vi "BRig_Host_formatData_test3_p2_subunit1.vi"(7 "input_filePath":string, 8 "input_error":errorcluster, 9 "input_data":u16[][](array[numeric]), 10 "input_headers":string[](array[string]), 11 "input_hdl_Workbooks":refnum<k7>) -> (0 "output_error":errorcluster, 3 "output_hdl_Worksbooks":refnum<k7>)   [LabVIEW 2014]
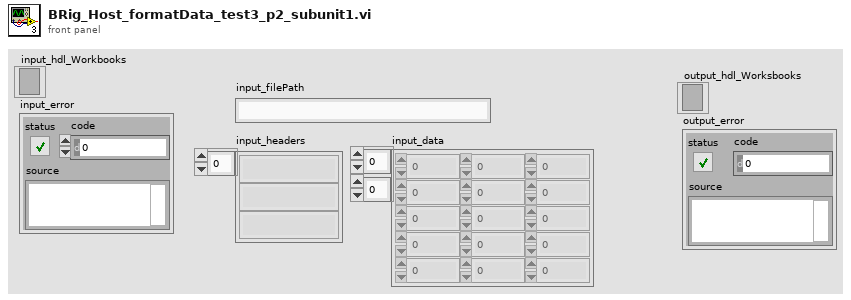
[diagram p1: front panel]
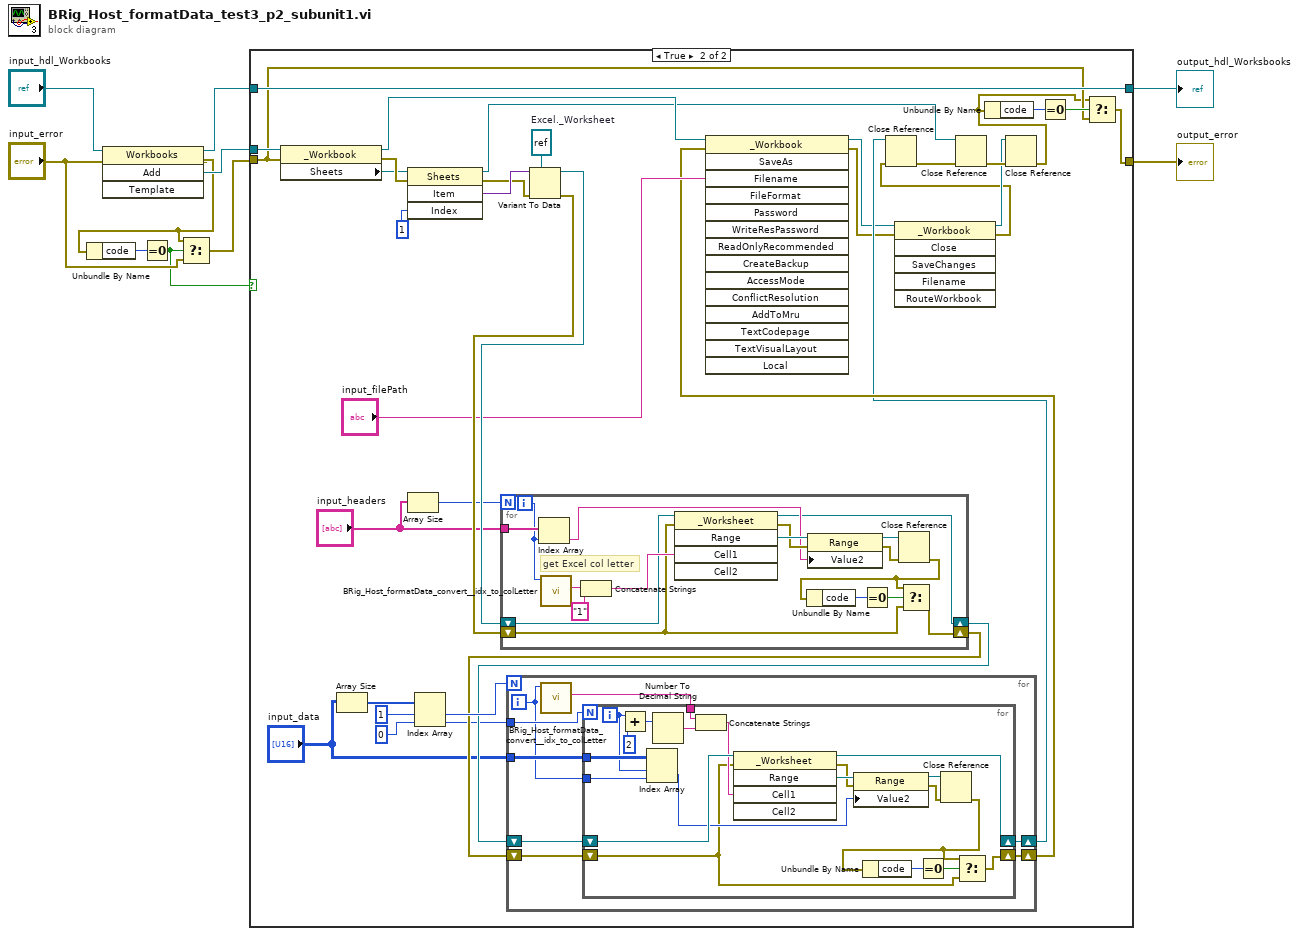
[diagram p0: block diagram]
diagram:
  n1 = invoke class="Workbooks" method="Add"(reference="input_hdl_Workbooks", error in="input_error") -> (reference out=w7:refnum<k7>, error out=w4:errorcluster, "Add"=w10:refnum<k7>)  [unwired: 2 in, 1 out]
  n2 = Unbundle By Name(w4) -> ("code"=w5:i32)
  n3 = Equal To 0?(x=w5) -> (x = 0?=w1:bool)
  n4 = Select(t=w4, s=w1, f="input_error") -> (s? t:f=w2:errorcluster)
  n5 = case shown="True" w1 {
    tunnel: w2 -> [w11 w15]
    tunnel: w10 -> [_ w46]
    tunnel: [w11 w14] -> w9
    tunnel: w7 -> [w12 w18]
    tunnel: [w12 w18] -> w6
    frame False {
    }
    frame True {
      w44 = refnum<k7> refnum  # Excel._Worksheet
      n6 = property class="_Workbook"(reference=w46, error in=w15) -> (reference out=w41:refnum<k7>, error out=w48:errorcluster, "Sheets"=w45:refnum<k7>)
      n7 = Array Size(array="input_data") -> (size(s)=w32:i32[])
      n8 = invoke class="Sheets" method="Item"(reference=w45, error in=w48, "Index"=1) -> (reference out=w40:refnum<k7>, error out=w42:errorcluster, "Item"=w43:variant)  [unwired: 1 in, 1 out]
      n9 = Array Size(array="input_headers") -> (size(s)=w33:i32)
      n10 = Index Array(array=w32, index #1=1 ("index"), index #2=0 ("index")) -> (element #1=w29:i32, element #2=w26:i32)
      n11 = Variant To Data(error in=w42, type=w44, Variant=w43) -> (data=w36:refnum<k7>, error out=w37:errorcluster)
      n12 = for {
        N: w33 -> [_]
        tunnel: "input_headers" -> [w93]
        shift-right: [w84] -> w27
        shift-left: w36 -> [w85]
        shift-right: [w77] -> w28
        shift-left: w37 -> [w78]
        i -> [w92]
        # "get Excel col letter"
        n13 = Index Array(array=w93, index=w92) -> (element=w86:string)
        n14 = call "BRig_Host_formatData_convert__idx_to_colLetter.vi"("input_idx"=w92) -> ("output_colLetter"=w90:string)  [unwired: 10 in]
        n15 = Concatenate Strings(w90, "1" ("string")) -> (w89:string)
        n16 = invoke class="_Worksheet" method="Range"(reference=w85, error in=w78, "Cell1"=w89) -> (reference out=w84:refnum<k7>, error out=w87:errorcluster, "Range"=w88:refnum<k7>)  [unwired: 2 in, 2 out]
        n17 = property class="Range"(reference=w88, error in=w87, "Value2"=w86) -> (reference out=w83:refnum<k7>, error out=w82:errorcluster)
        n18 = Close Reference(reference=w83, error in (no error)=w82) -> (error out=w79:errorcluster)
        n19 = Unbundle By Name(w79) -> ("code"=w81:i32)
        n20 = Equal To 0?(x=w81) -> (x = 0?=w80:bool)
        n21 = Select(t=w79, s=w80, f=w78) -> (s? t:f=w77:errorcluster)
      }
      n22 = for {
        N: w29 -> [_]
        shift-right: [w50] -> w24
        shift-left: w28 -> [w56]
        shift-right: [w49] -> w23
        shift-left: w27 -> [w55]
        tunnel: w26 -> [w54]
        tunnel: "input_data" -> [w52]
        i -> [w51]
        n23 = call "BRig_Host_formatData_convert__idx_to_colLetter.vi"("input_idx"=w51) -> ("output_colLetter"=w53:string)  [unwired: 10 in]
        n24 = for {
          N: w54 -> [_]
          shift-right: [w57] -> w50
          shift-left: w56 -> [w58]
          shift-right: [w62] -> w49
          shift-left: w55 -> [w69]
          tunnel: w53 -> [w73]
          tunnel: w52 -> [w72]
          tunnel: w51 -> [w70]
          i -> [w71]
          n25 = Add(x=w71, y=2 ("string")) -> (x+y=w75:i32)
          n26 = Index Array(array=w72, index (row)=w71, index (col)=w70) -> (element=w65:u16)
          n27 = Number To Decimal String(number=w75) -> (decimal integer string=w74:string)  [unwired: 1 in]
          n28 = Concatenate Strings(w73, w74) -> (w68:string)
          n29 = invoke class="_Worksheet" method="Range"(reference=w69, error in=w58, "Cell1"=w68) -> (reference out=w62:refnum<k7>, error out=w66:errorcluster, "Range"=w67:refnum<k7>)  [unwired: 2 in, 2 out]
          n30 = property class="Range"(reference=w67, error in=w66, "Value2"=w65) -> (reference out=w64:refnum<k7>, error out=w63:errorcluster)
          n31 = Close Reference(reference=w64, error in (no error)=w63) -> (error out=w59:errorcluster)
          n32 = Unbundle By Name(w59) -> ("code"=w61:i32)
          n33 = Equal To 0?(x=w61) -> (x = 0?=w60:bool)
          n34 = Select(t=w59, s=w60, f=w58) -> (s? t:f=w57:errorcluster)
        }
      }
      n35 = invoke class="_Workbook" method="SaveAs"(reference=w41, error in=w24, "Filename"="input_filePath") -> (reference out=w21:refnum<k7>, error out=w22:errorcluster)  [unwired: 12 in, 13 out]
      n36 = invoke class="_Workbook" method="Close"(reference=w21, error in=w22) -> (reference out=w20:refnum<k7>, error out=w19:errorcluster)  [unwired: 4 in, 4 out]
      n37 = Close Reference(reference=w23, error in (no error)=w19) -> (error out=w39:errorcluster)
      n38 = Close Reference(reference=w40, error in (no error)=w39) -> (error out=w38:errorcluster)
      n39 = Close Reference(reference=w20, error in (no error)=w38) -> (error out=w13:errorcluster)
      n40 = Unbundle By Name(w13) -> ("code"=w17:i32)
      n41 = Equal To 0?(x=w17) -> (x = 0?=w16:bool)
      n42 = Select(t=w13, s=w16, f=w15) -> (s? t:f=w14:errorcluster)
    }
  }
  "output_hdl_Worksbooks" <- w6
  "output_error" <- w9
